vi "判定测试.vi"() -> ()   [LabVIEW 2019]
uses:
  <userlib>/_MGI/1D Array/MGI Running Average/MGI Running Average(DBL).vi
panel:
  out "曲线判定结果":T1(array[cluster])
  out "XY图":cluster{dbl[], dbl[]}[](graph)
  in  "曲线判定条件":T2(array[cluster])
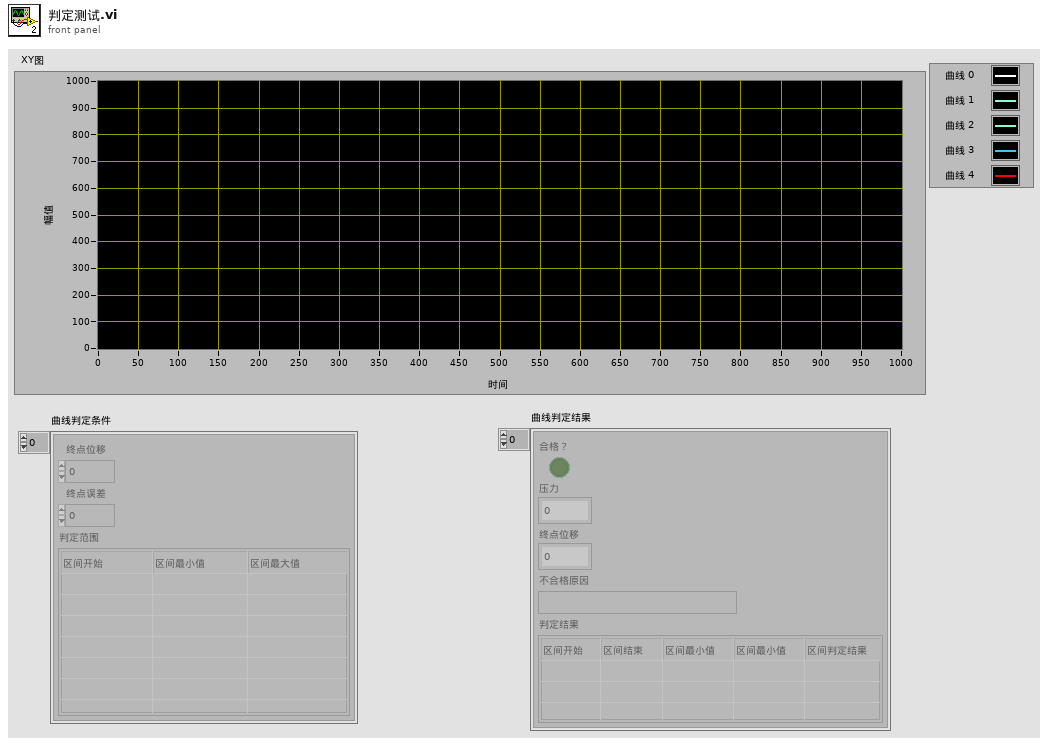
[diagram p1: front panel]
types:
  T1 = cluster{"合格？":bool, "压力":dbl, "终点位移":dbl, "不合格原因":string, "判定结果":string[][]}[]
  T2 = cluster{"终点位移":dbl, "终点误差":dbl, "判定范围":string[][]}[]
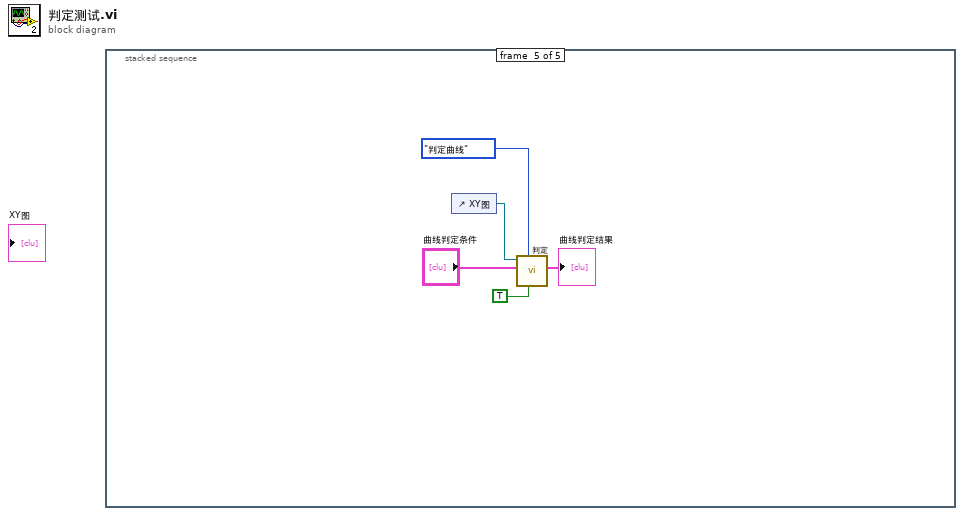
[diagram p0: block diagram]
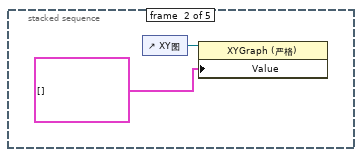
[diagram p3: hidden frame]
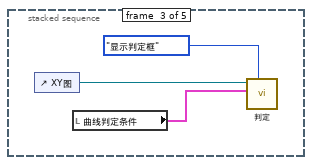
[diagram p4: hidden frame]
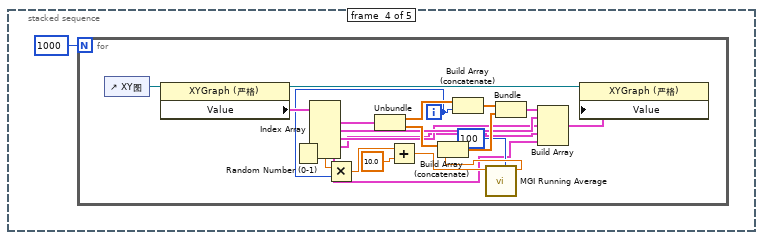
[diagram p5: hidden frame]
diagram:
  n1 = stacked-sequence {
    frame #0 {
    }
    frame #1 {
      n2 = control-ref of="XY图"() -> (w2:refnum<vi>)
      n3 = property class="XYGraph (严格)"(reference=w2, "Value"=cluster{dbl[], dbl[]}[] []) -> ()  [unwired: 1 in, 2 out]
    }
    frame #2 {
      n4 = control-ref of="XY图"() -> (w5:refnum<vi>)
      n5 = local read "曲线判定条件"() -> (w3:T2)
      n6 = call "判定.vi"("方式"=enum16{"清除曲线", "显示判定框", "判定曲线"}."显示判定框", "曲线判定条件"=w3, "曲线引用"=w5) -> ()  [unwired: 6 in, 3 out]
    }
    frame #3 {
      n7 = for {
        N: 1000 -> [_]
        i -> [w11]
        n8 = control-ref of="XY图"() -> (w27:refnum<vi>)
        n9 = property class="XYGraph (严格)"(reference=w27) -> (reference out=w15:refnum<vi>, "Value"=w26:cluster{dbl[], dbl[]}[])  [unwired: 1 in, 1 out]
        n10 = Random Number (0-1)() -> (number: 0 to 1=w22:dbl)
        n11 = Index Array(array=w26) -> (element #1=w25:cluster{dbl[], dbl[]}, element #2=w14:cluster{dbl[], dbl[]}, element #3=w13:cluster{dbl[], dbl[]}, element #4=w12:cluster{dbl[], dbl[]}, element #5=w7:cluster{dbl[], dbl[]})  [unwired: 5 in]
        n12 = Multiply(x=w22, y=w11) -> (x*y=w21:dbl)
        n13 = Unbundle(w25) -> (w24:dbl[], w23:dbl[])
        n14 = Add(x=w21, y=10.0) -> (x+y=w10:dbl)
        n15 = Build Array (concatenate)(w24, w11) -> (w19:dbl[])
        n16 = call-poly <userlib>:"MGI Running Average.vi"("Averaging Size"=100, "Value"=w10) -> ("Average"=w9:dbl)  [unwired: 9 in]
        n17 = Build Array (concatenate)(w23, w9) -> (w18:dbl[])
        n18 = Bundle(w19, w18) -> (w17:cluster{dbl[], dbl[]})  [unwired: 1 in]
        n19 = Build Array(w17, w14, w13, w12, w7) -> (w16:cluster{dbl[], dbl[]}[])
        n20 = property class="XYGraph (严格)"(reference=w15, "Value"=w16) -> ()  [unwired: 1 in, 2 out]
      }
    }
    frame #4 {
      n21 = control-ref of="XY图"() -> (w31:refnum<vi>)
      n22 = call "判定.vi"("显示超限点"=TRUE, "方式"=enum16{"清除曲线", "显示判定框", "判定曲线"}."判定曲线", "曲线判定条件"="曲线判定条件", "曲线引用"=w31) -> ("曲线判定结果"=→"曲线判定结果":T1)  [unwired: 5 in, 2 out]
    }
  }
